vi "Generate Patch Seq Img Core.vi"(0 "tdms file ref":refnum<k34>, 1 "Channel to process":enum16{"Red", "Green"}(ring), 5 "All header parameters":T1={"Imaging Protocol"=enum."AOL Z-Stack", "Number of POI"=0, "Number of Miniscans"=0, "Number of Trials"=0, "Number of Cycles "=0, "# Averaged Frames"=0, "Laser power (%)"=0, "Pockels"=0.0, "Acquisition Length (sec)"=0.0, "Fill time (us)"=0.0, "POI Dwell time (us)"=0.0, "Miniscan Dwell time per pixel (us)"=0.0, "PMT 1"=0.0, "PMT 2"=0.0, "Back Apperture"=0.0, "Zoom"=0.0, "Frame Size"=200, "Center Frequency"=0.0, "Field of View"=0.0, "DwellTime (us)"=0.0, "Wavelength (nm)"=0.0, "AOL Z"=0.0, "AOL Mode"=enum."Raster", "GridXY"=0.0, "GridZ"=0.0, "TriggerDelay (sec)"=0.0, "Number of Pixels in Miniscan"=0, "Experiment folder path"=path "", "X centre"=0.0, "Y centre"=0.0, "Angle (degrees)"=0.0, "Plane Mode"=0, "Software version"=0.0, "Objective"="Olympus  20X", "MotorZ Calibration"=0, "Pockels Calibration"=0, "Threshold"=[], "Video length (sec)"=0.0, "Frame rate (fps)"=0, "Rectangle ROI length (pixels)"=0, "Rectangle ROI height (pixels)"=0} {"Pockels" format="%#.6g"; "Software version" format="%#.6g"; "Plane Mode" items=["XY Plane"]; "Angle (degrees)" format="%#.6g"; "Frame Size" items=["100X100"=100, "128X128"=128, "200X200"=200, "256X256"=256, "512X512"=512, "1024x1024"=1024, "2048x2048"=2048]; "Back Apperture" format="%#.6g"; "PMT 2" format="%#.6g"; "PMT 1" format="%#.6g"; "Miniscan Dwell time per pixel (us)" format="%#.6g"; "Zoom" format="%#.6g"; "POI Dwell time (us)" format="%#.6g"; "Acquisition Length (sec)" format="%#.6g"; "Fill time (us)" format="%#.6g"}, 7 "TDMS file path & name":path=path "C:/Users/Theo/Desktop/Datasets/140401_17_44_08-rig 3 debugging/Functional imaging TDMS data files/001.tdms", 9 "Patch Image Folder":path[](array[path]), 11 "error in (no error)":errorcluster, 13 "TIFF file handles":i32[](array[numeric]), 14 "Trial Number":i32) -> (4 "tdms file out":refnum<k34>, 15 "error out":errorcluster)   [LabVIEW 2013]
uses:
  User Interface/Visualisation/Functional Imaging Viewer/SubVIs/Experiment header interface/Typedefs/Header parameters cluster-ALL.ctl
  Typedefs/Imaging Protocols enum.ctl
  Typedefs/Frame Size.ctl
  Typedefs/AOL modes.ctl
  Typedefs/Plane Mode.ctl
  Typedefs/Objective selector control enum.ctl
  Typedefs/Channel Selector.ctl
  Globals/gl_funct TIFF export globals.vi
  <vilib>/vision/NI_Vision_Development_Module.lvlib
panel:
  out "Loop time (ms)":u32
  # "Re-entrant"
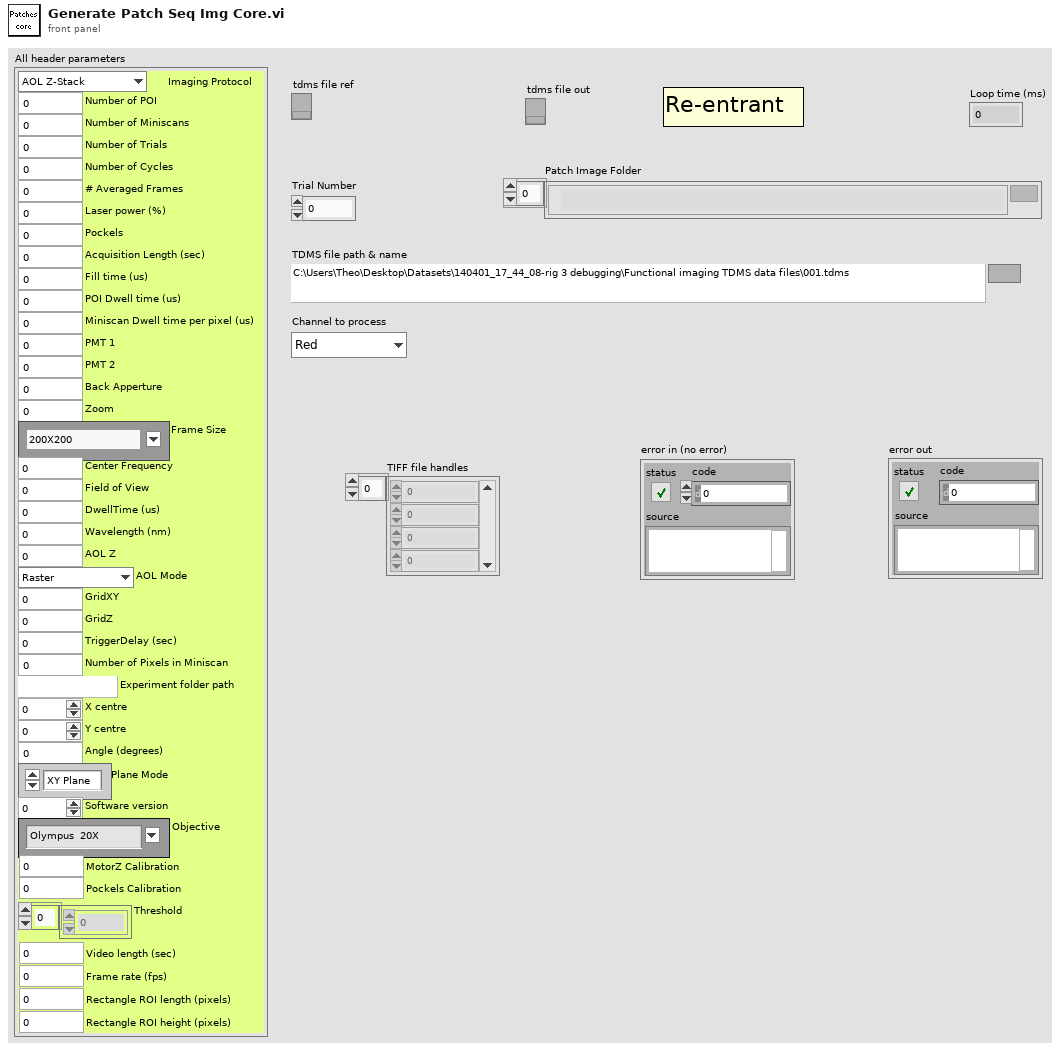
[diagram p1: front panel]
types:
  T1 = typedef "Header parameters cluster-ALL.ctl" = cluster{"Imaging Protocol":T2, "Number of POI":u16, "Number of Miniscans":u16, "Number of Trials":u16, "Number of Cycles ":u64, "# Averaged Frames":u16, "Laser power (%)":u8, "Pockels":dbl, "Acquisition Length (sec)":dbl, "Fill time (us)":dbl, "POI Dwell time (us)":dbl, "Miniscan Dwell time per pixel (us)":dbl, "PMT 1":dbl, "PMT 2":dbl, "Back Apperture":dbl, "Zoom":dbl, "Frame Size":T3, "Center Frequency":dbl, "Field of View":dbl, "DwellTime (us)":dbl, "Wavelength (nm)":dbl, "AOL Z":dbl, "AOL Mode":T4, "GridXY":dbl, "GridZ":dbl, "TriggerDelay (sec)":dbl, "Number of Pixels in Miniscan":u16, "Experiment folder path":path, "X centre":dbl, "Y centre":dbl, "Angle (degrees)":dbl, "Plane Mode":T5, "Software version":dbl, "Objective":T6, "MotorZ Calibration":u32, "Pockels Calibration":u32, "Threshold":u16[], "Video length (sec)":dbl, "Frame rate (fps)":u8, "Rectangle ROI length (pixels)":u16, "Rectangle ROI height (pixels)":u16}
  T2 = typedef "Imaging Protocols enum.ctl" = enum16{"AOL Z-Stack", "Motor Z Stack", "Functional Acquisition", "Single Plane Acquisition", "Volume Acquisition", "Live Imaging", "Live Plane Imaging", "Live Volume Imaging"}
  T3 = typedef "Frame Size.ctl" = u16
  T4 = typedef "AOL modes.ctl" = enum16{"Raster", "Structural", "Pointing", "Mini Scan", "Alignment"}
  T5 = typedef "Plane Mode.ctl" = u16
  T6 = typedef "Objective selector control enum.ctl" = string
  T7 = typedef "Funct TIFF exporter ctrl refs.ctl" = cluster{"This VI":refnum<vi>, "Current Experiment":refnum<vi>, "Imaging protocol":refnum<vi>, "Predominant ROI type":refnum<vi>, "Patches in Experiment":refnum<vi>, "Folder Path":refnum<vi>, "Export":refnum<vi>, "Trial number":refnum<vi>, "Output TIFF type":refnum<vi>}
  T8 = typedef "Exported TIFF type.ctl" = enum16{"One multi-page TIFF file for each rectangle", "Individual TIFF files"}
  T9 = typedef "Channel Selector.ctl" = enum16{"Red Channel", "Green Channel", "Blended"}
  T10 = cluster{"Number of cycles":i32, "number of planes":i32, "number of miniscans in a Plane":i32, "number of pixels in a miniscan":i32}
  T11 = typedef "Image Type" = u32
  T12 = typedef "IMAQ Image.ctl" = refnum<image>
  T13 = typedef "IMAQ AVI2 Refnum.ctl" = refnum<k20>
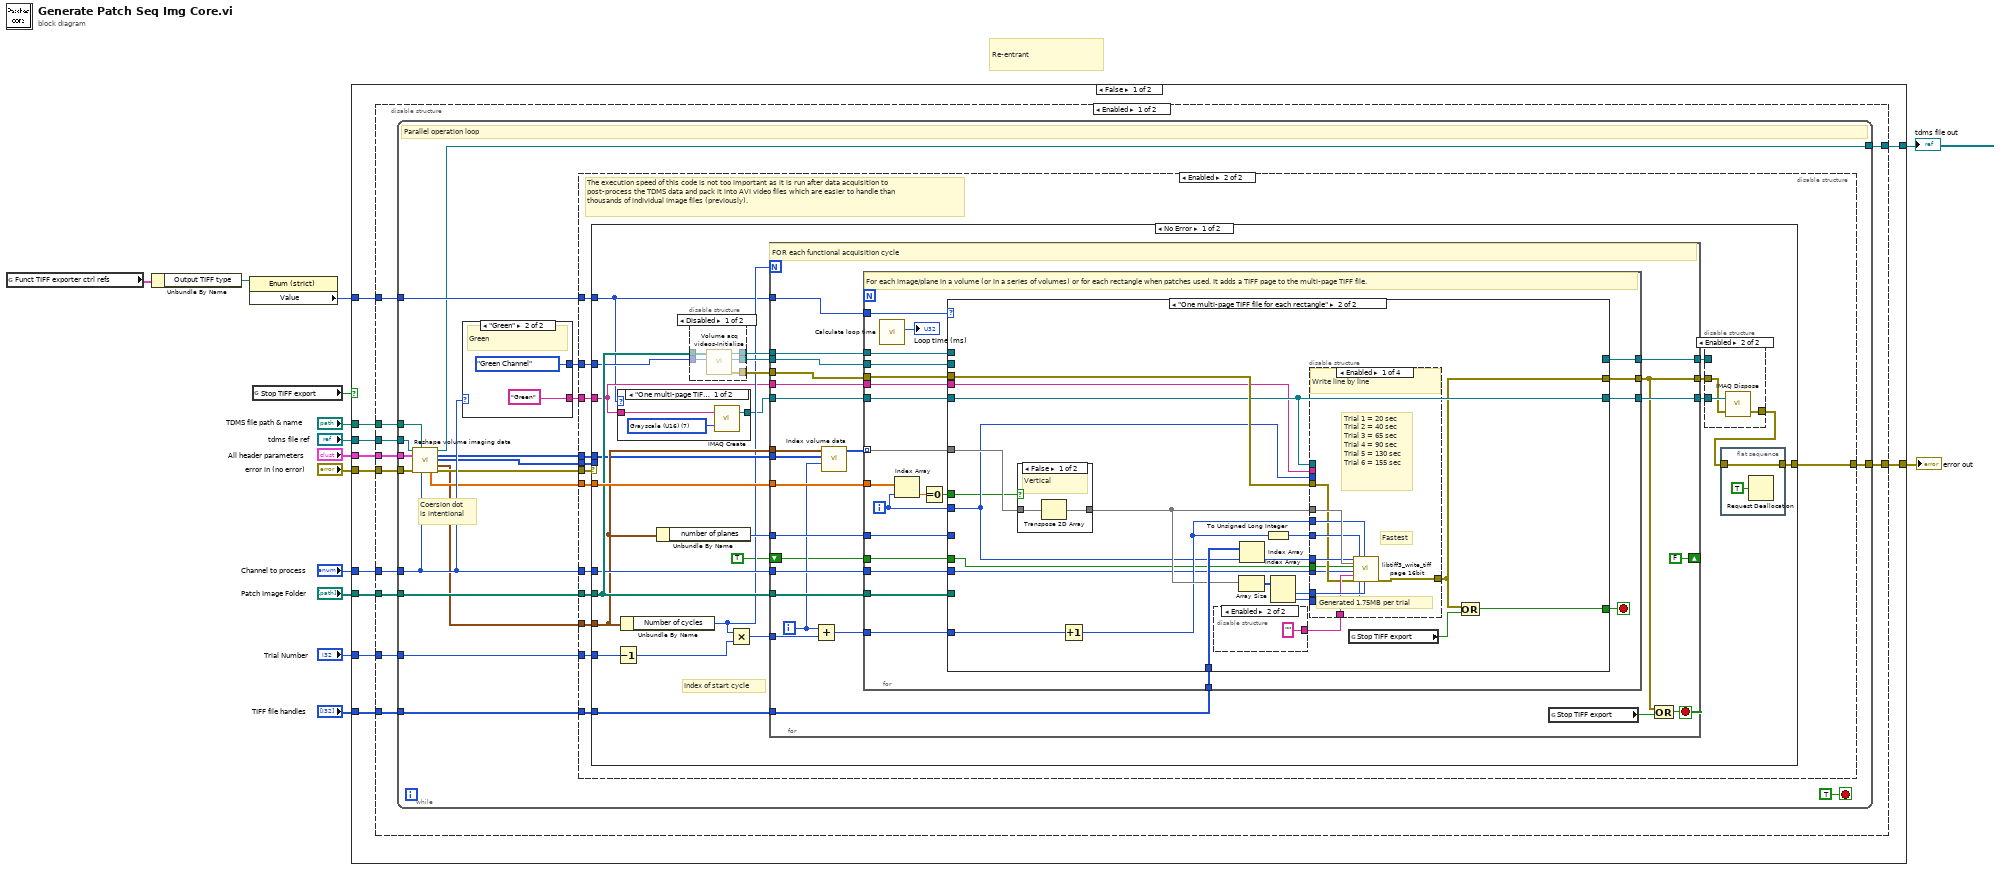
[diagram p0: block diagram]
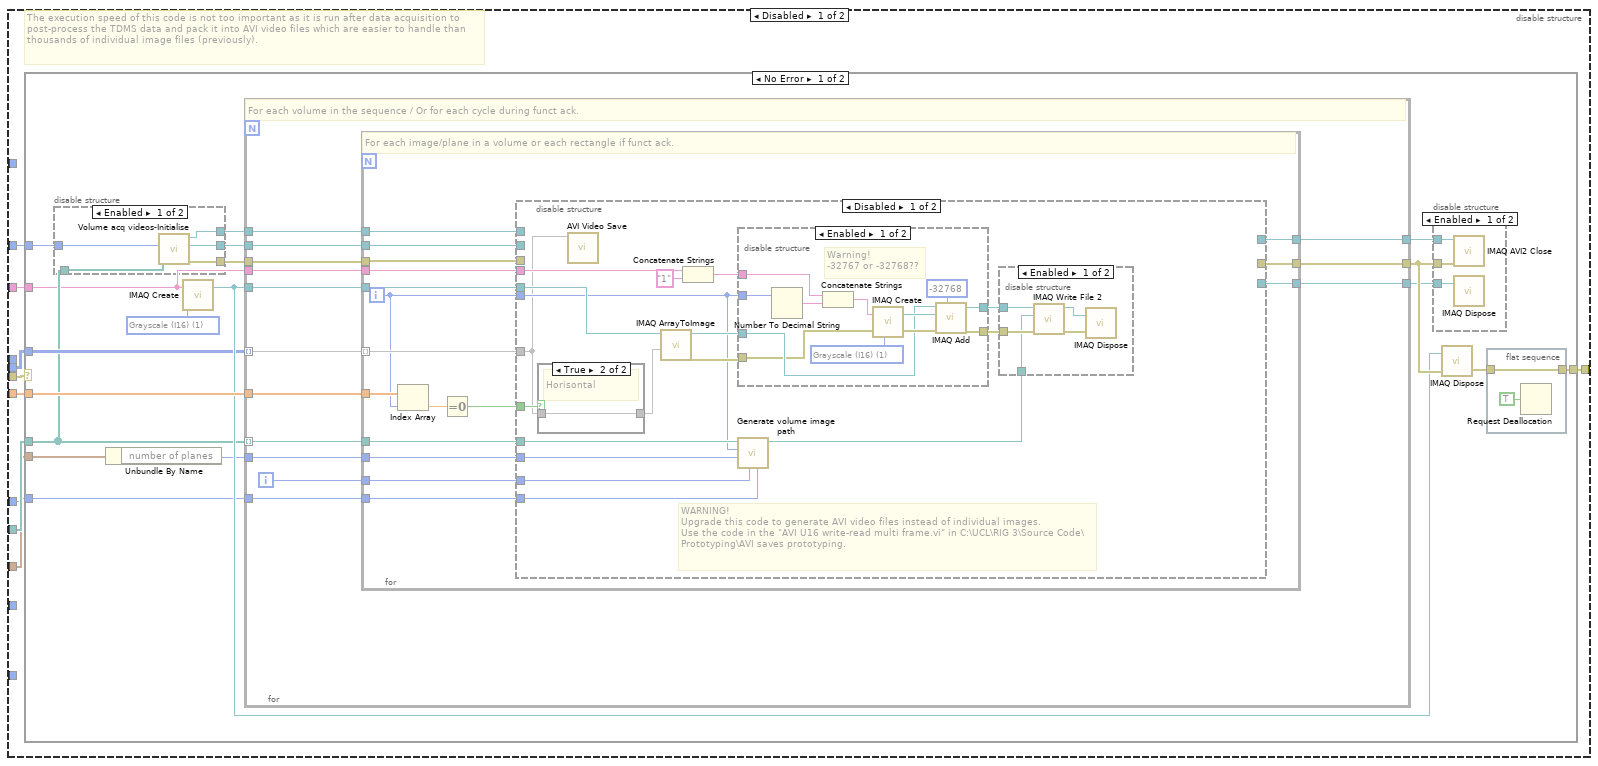
[diagram p2: hidden frame]
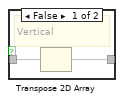
[diagram p5: hidden frame]
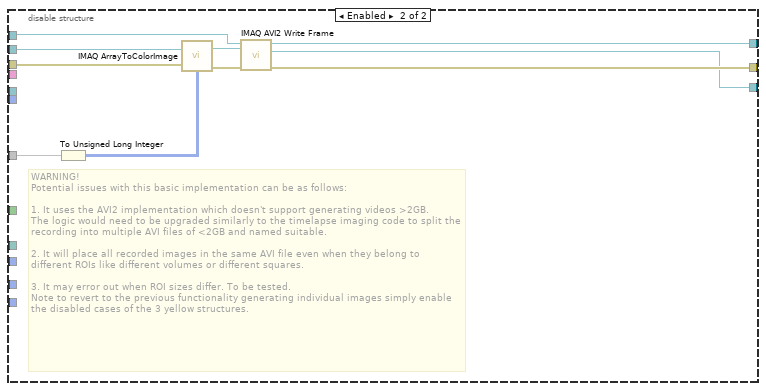
[diagram p8: hidden frame]
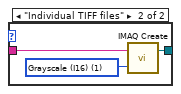
[diagram p10: hidden frame]
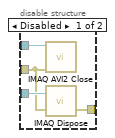
[diagram p12: hidden frame]
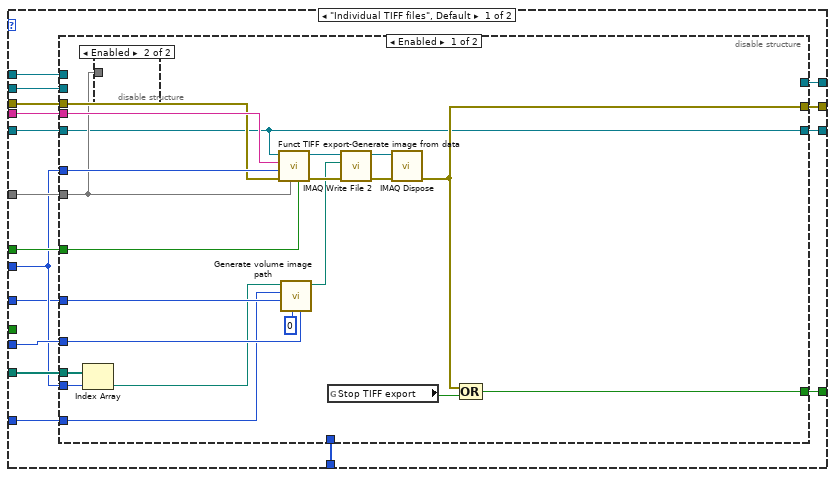
[diagram p13: hidden frame]
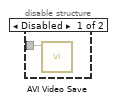
[diagram p14: hidden frame]
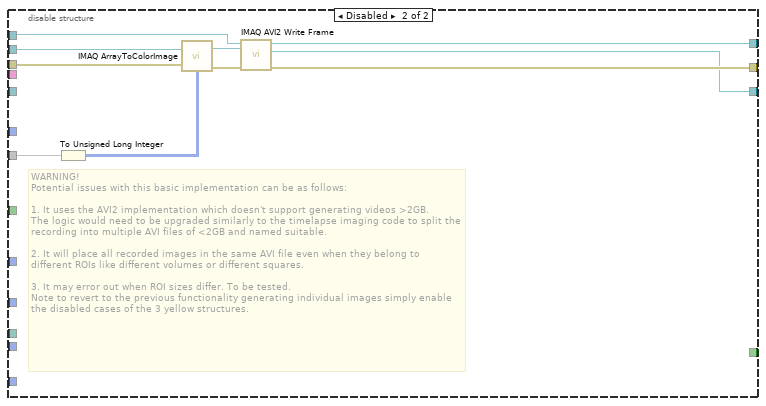
[diagram p15: hidden frame]
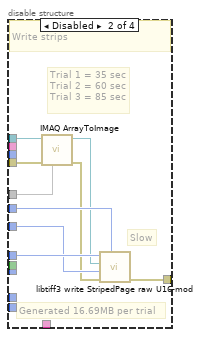
[diagram p16: hidden frame]
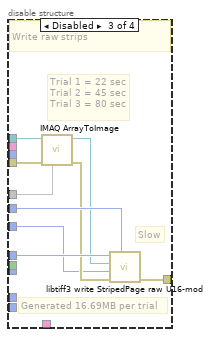
[diagram p17: hidden frame]
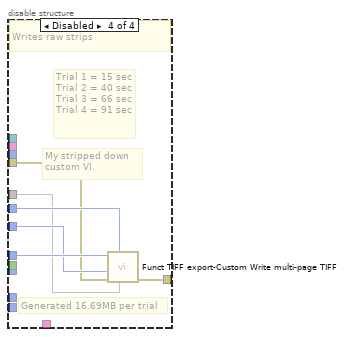
[diagram p18: hidden frame]
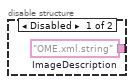
[diagram p19: hidden frame]
diagram:
  # "Re-entrant"
  n1 = global read "gl_funct TIFF export globals.vi" "Funct TIFF exporter ctrl refs"() -> (w6:T7)
  n2 = Unbundle By Name(w6) -> ("Output TIFF type"=w7:refnum<vi>)
  n3 = property on="Property Node" class="Enum (strict)"(reference=w7) -> ("Value"=w5:T8)  [unwired: 1 in, 2 out]
  n4 = global read "gl_funct TIFF export globals.vi" "Stop TIFF export"() -> (w10:bool)
  n5 = case shown="False" w10 {
    tunnel: [w25 w528] -> w14
    tunnel: "error in (no error)" -> [w24 w528]
    tunnel: "Channel to process" -> [w23 _]
    tunnel: "Patch Image Folder" -> [w22 _]
    tunnel: "Trial Number" -> [w21 _]
    tunnel: "TIFF file handles" -> [w20 _]
    tunnel: w5 -> [w19 _]
    tunnel: "tdms file ref" -> [w18 w527]
    tunnel: "All header parameters" -> [w17 _]
    tunnel: "TDMS file path & name" -> [w16 _]
    tunnel: [w15 w527] -> w1
    frame False {
      n6 = disable-structure shown="Enabled" {
        disable-tunnel: [w36 w399] -> w25
        disable-tunnel: w22 -> [w35 w398]
        disable-tunnel: w24 -> [w34 w397]
        disable-tunnel: w23 -> [w33 w396]
        disable-tunnel: w21 -> [w32 _]
        disable-tunnel: w20 -> [w31 _]
        disable-tunnel: w19 -> [w30 _]
        disable-tunnel: w18 -> [w29 w394]
        disable-tunnel: w17 -> [w28 w393]
        disable-tunnel: w16 -> [w27 w395]
        disable-tunnel: [w26 w392] -> w15
        frame Enabled {
          n7 = while {
            tunnel: [w55] -> w36
            tunnel: w35 -> [w54]
            tunnel: w34 -> [w53]
            tunnel: w33 -> [w52]
            tunnel: w32 -> [w51]
            tunnel: w31 -> [w50]
            tunnel: w30 -> [w49]
            tunnel: w29 -> [w38]
            tunnel: w28 -> [w41]
            tunnel: w27 -> [w40]
            tunnel: [w39] -> w26
            stop <- TRUE stop-if-true
            # "Coersion dot\nis intentional"
            # "Parallel operation loop"
            n8 = call "Reshape volume imaging data.vi"("tdms file ref"=w38, "TDMS file path & name"=w40, "All header parameters"=w41, "error in (no error)"=w53, "Channel to process"=w52) -> ("tdms file out"=w39:refnum<k34>, "Single channel data"=w43:u16[], "Channel 4D data"=w42:u16[][][][], "Volumetric parameters"=w44:T10, "Angles (deg)"=w45:dbl[], "error out"=w47:errorcluster)  [unwired: 5 in]
            n9 = case shown="\"Green\"" w52 {
              tunnel: ["Red" ("Image Name") "Green" ("Image Name")] -> w48
              tunnel: [Channel_Selector."Red Channel" ("Channel") Channel_Selector."Green Channel" ("Channel")] -> w46
              frame "Red", Default {
                # "Red"
              }
              frame "Green" {
                # "Green"
              }
            }
            n10 = disable-structure shown="Enabled" {
              disable-tunnel: [w64 w186] -> w55
              disable-tunnel: w54 -> [w63 w185]
              disable-tunnel: w48 -> [w62 w184]
              disable-tunnel: w42 -> [w61 w183]
              disable-tunnel: w47 -> [w60 w182]
              disable-tunnel: w46 -> [w59 w181]
              disable-tunnel: w45 -> [w58 w180]
              disable-tunnel: w52 -> [w57 w179]
              disable-tunnel: w44 -> [w56 w178]
              disable-tunnel: w43 -> [_ w177]
              disable-tunnel: w51 -> [_ w175]
              disable-tunnel: w50 -> [_ w176]
              disable-tunnel: w49 -> [_ w174]
              frame Disabled {
                # "The execution speed of this code is not too important as it is run after data acquisition to post-process the TDMS data and pack it into AVI video files which are easier to handle than thousands of individual image files (previously)."
                n11 = case shown="No Error" w60 {
                  selector: w60 -> [_ w173]
                  tunnel: [w68 w173] -> w64
                  tunnel: w58 -> [w82 _]
                  tunnel: w61 -> [w74 _]
                  tunnel: w56 -> [w65 _]
                  tunnel: w63 -> [w71 _]
                  tunnel: w62 -> [w70 _]
                  tunnel: w57 -> [w67 _]
                  tunnel: w59 -> [w66 _]
                  frame No Error {
                    w73 = T11 1 items=["Grayscale (U8)", "Grayscale (I16)", "Grayscale (SGL)", "Complex (CSG)", "RGB (U32)", "HSL (U32)", "RGB (U64)", "Grayscale (U16)"] ("Image Type")
                    n12 = disable-structure "Diagram Disable Structure" shown="Enabled" {
                      disable-tunnel: [w89 _] -> w75
                      disable-tunnel: [w88 _] -> w76
                      disable-tunnel: [w87 _] -> w77
                      disable-tunnel: w71 -> [w86 _]
                      disable-tunnel: w66 -> [w85 _]
                      frame Enabled {
                        n13 = call "Volume acq videos-Initialise.vi"("Channel"=w85, "created path"=w86) -> ("error out"=w89:errorcluster, "Temp Image"=w88:T12, "Refnum out"=w87:T13)  [unwired: 7 in]
                      }
                      frame Disabled {
                      }
                    }
                    n14 = Unbundle By Name(w65) -> ("number of planes"=w72:i32)
                    n15 = call "IMAQ Create"("Image Name"=w70, "Image Type"=w73) -> ("New Image"=w80:T12)  [unwired: 3 in, 1 out]
                    n16 = for {
                      tunnel: w74 -> [w106] mode=indexing
                      tunnel: w80 -> [w105]
                      tunnel: w71 -> [w104] mode=indexing
                      tunnel: w72 -> [w102]
                      tunnel: w76 -> [w101]
                      tunnel: w77 -> [w100]
                      tunnel: w75 -> [w99]
                      tunnel: [w98] -> w81
                      tunnel: [w97] -> w78
                      tunnel: [w96] -> w79
                      tunnel: w82 -> [w95]
                      tunnel: w70 -> [w94]
                      tunnel: w67 -> [w93]
                      i -> [w103]
                      # "For each volume in the sequence / Or for each cycle during funct ack."
                      n17 = for {
                        tunnel: w106 -> [w110] mode=indexing
                        tunnel: w105 -> [w123]
                        tunnel: w104 -> [w122]
                        tunnel: w103 -> [w121]
                        tunnel: w102 -> [w120]
                        tunnel: w101 -> [w118]
                        tunnel: w100 -> [w119]
                        tunnel: w99 -> [w117]
                        tunnel: [w116] -> w98
                        tunnel: [w115] -> w97
                        tunnel: [w114] -> w96
                        tunnel: w95 -> [w109]
                        tunnel: w94 -> [w112]
                        tunnel: w93 -> [w111]
                        i -> [w108]
                        # "For each image/plane in a volume or each rectangle if funct ack."
                        n18 = Index Array(array=w109, index=w108) -> (element=w107:dbl)
                        n19 = Equal To 0?(x=w107) -> (x = 0?=w113:bool)
                        n20 = disable-structure shown="Disabled" {
                          disable-tunnel: w123 -> [w140 _]
                          disable-tunnel: w122 -> [w135 _]
                          disable-tunnel: w121 -> [w133 _]
                          disable-tunnel: w120 -> [w132 _]
                          disable-tunnel: w108 -> [w131 _]
                          disable-tunnel: w119 -> [_ w169]
                          disable-tunnel: w118 -> [_ w168]
                          disable-tunnel: w117 -> [_ w167]
                          disable-tunnel: [_ w166] -> w116
                          disable-tunnel: [_ w165] -> w115
                          disable-tunnel: [_ w164] -> w114
                          disable-tunnel: w113 -> [w130 _]
                          disable-tunnel: w110 -> [w125 w163]
                          disable-tunnel: w112 -> [w128 _]
                          disable-tunnel: w111 -> [w124 _]
                          frame Disabled {
                            # "WARNING!\nUpgrade this code to generate AVI video files instead of individual images.\nUse the code in the \"AVI U16 write-read multi frame.vi\" in C:\\UCL\\RIG 3\\Source Code\\Prototyping\\AVI saves prototyping."
                            n21 = case shown="True" w130 {
                              tunnel: w125 -> [w142 w143]
                              tunnel: [w141 w143] -> w129
                              frame False {
                                # "Vertical"
                                n22 = Transpose 2D Array(2D array=w142) -> (transposed array=w141:u16[][])
                              }
                              frame True {
                                # "Horisontal"
                              }
                            }
                            n23 = call "AVI Video Save.vi"("Image Pixels"=w125) -> ()  [unwired: 9 in, 2 out]
                            n24 = call "IMAQ ArrayToImage"("Image Pixels (I16)"=w129, "Image"=w140) -> ("error out"=w136:errorcluster, "Image Out"=w139:T12)  [unwired: 8 in]
                            n25 = Concatenate Strings(w128, "1" ("string")) -> (w126:string)
                            n26 = call "Generate volume image path.vi"("Channel to process"=w124, "Volume index"=w133, "Number of planes"=w132, "Plane index (within its volume)"=w131, "Folder path"=w135) -> ("File path"=w134:path)  [unwired: 5 in, 1 out]
                            n27 = disable-structure shown="Enabled" {
                              disable-tunnel: w131 -> [w154 _]
                              disable-tunnel: w139 -> [w153 w162]
                              disable-tunnel: [w152 w162] -> w138
                              disable-tunnel: [w150 w161] -> w137
                              disable-tunnel: w136 -> [w151 w161]
                              disable-tunnel: w126 -> [w149 _]
                              frame Enabled {
                                w156 = T11 1 items=["Grayscale (U8)", "Grayscale (I16)", "Grayscale (SGL)", "Complex (CSG)", "RGB (U32)", "HSL (U32)", "RGB (U64)"] ("Image Type")
                                # "Warning!\n-32767 or -32768??"
                                n28 = Number To Decimal String(number=w154) -> (decimal integer string=w157:string)  [unwired: 1 in]
                                n29 = Concatenate Strings(w149, w157) -> (w158:string)
                                n30 = call "IMAQ Create"("Image Name"=w158, "Image Type"=w156, "error in (no error)"=w151) -> ("New Image"=w159:T12, "error out"=w160:errorcluster)  [unwired: 2 in]
                                n31 = call "IMAQ Add"("Image Src A"=w153, "Constant"=i16 -32768, "Image Dst"=w159, "error in (no error)"=w160) -> ("Image Dst Out"=w152:T12, "error out"=w150:errorcluster)  [unwired: 3 in]
                              }
                              frame Disabled {
                              }
                            }
                            n32 = disable-structure shown="Enabled" {
                              disable-tunnel: w138 -> [w146 _]
                              disable-tunnel: w137 -> [w145 _]
                              disable-tunnel: w134 -> [w144 _]
                              frame Enabled {
                                n33 = call-poly "IMAQ Write File 2"("error in (no error)"=w145, "File Path"=w144, "Image"=w146) -> ("error out"=w148:errorcluster, "Image Out (duplicate)"=w147:T12)  [unwired: 7 in]
                                n34 = call "IMAQ Dispose"("Image"=w147, "error in (no error)"=w148) -> ()  [unwired: 4 in, 1 out]
                              }
                              frame Disabled {
                              }
                            }
                          }
                          frame Enabled {
                            # "WARNING!\nPotential issues with this basic implementation can be as follows:\n\n1. It uses the AVI2 implementation which doesn't support generating videos >2GB. \nThe logic would need to be upgraded similarly to the timelapse imaging code to split the recording into multiple AVI files of <2GB and named suitable.\n\n2. It will place all recorded images in the same AVI file even when they belong to different ROIs like different volumes or different squares.\n\n3. It may error out when ROI sizes differ. To be tested.\nNote to revert to the previous functionality generating individual images simply enable the disabled cases of the 3 yellow structures."
                            n35 = To Unsigned Long Integer(number=w163) -> (unsigned 32bit integer=w171:u32[][])
                            n36 = call "IMAQ ArrayToColorImage"("Image Pixels (U32)"=w171, "Image"=w168, "error in (no error)"=w167) -> ("Image Out"=w172:T12, "error out"=w170:errorcluster)  [unwired: 1 in, 1 out]
                            n37 = call "IMAQ AVI2 Write Frame"("error in (no error)"=w170, "Image"=w172, "AVI Refnum"=w169) -> ("error out"=w166:errorcluster, "Image Out (duplicate)"=w164:T12, "AVI Refnum (duplicate)"=w165:T13)  [unwired: 6 in]
                          }
                        }
                      }
                    }
                    n38 = disable-structure "Diagram Disable Structure" shown="Enabled" {
                      disable-tunnel: w78 -> [w92 _]
                      disable-tunnel: w81 -> [w91 _]
                      disable-tunnel: w79 -> [w90 _]
                      frame Enabled {
                        n39 = call "IMAQ AVI2 Close"("error in (no error)"=w91, "AVI Refnum"=w92) -> ()  [unwired: 9 in, 1 out]
                        n40 = call "IMAQ Dispose"("Image"=w90) -> ()  [unwired: 5 in, 1 out]
                      }
                      frame Disabled {
                      }
                    }
                    n41 = call "IMAQ Dispose"("Image"=w80, "error in (no error)"=w81) -> ("error out"=w69:errorcluster)  [unwired: 4 in]
                    n42 = flat-sequence {
                      tunnel: w69 -> [w83]
                      tunnel: [w83] -> w68
                      frame #0 {
                        n43 = Request Deallocation(TRUE ("flag")) -> ()
                      }
                    }
                  }
                  frame Error {
                  }
                }
              }
              frame Enabled {
                # "The execution speed of this code is not too important as it is run after data acquisition to post-process the TDMS data and pack it into AVI video files which are easier to handle than thousands of individual image files (previously)."
                n44 = case shown="No Error" w182 {
                  selector: w182 -> [_ w387]
                  tunnel: [w202 w387] -> w186
                  tunnel: w180 -> [w210 _]
                  tunnel: w183 -> [_ _]
                  tunnel: w178 -> [w199 _]
                  tunnel: w185 -> [w203 _]
                  tunnel: w184 -> [w190 _]
                  tunnel: w179 -> [w201 _]
                  tunnel: w181 -> [w200 _]
                  tunnel: w177 -> [w198 _]
                  tunnel: w175 -> [w196 _]
                  tunnel: w176 -> [w195 _]
                  tunnel: w174 -> [w188 _]
                  frame No Error {
                    # "Index of start cycle"
                    n45 = Decrement(x=w196) -> (x-1=w194:i32)
                    n46 = case shown="\"One multi-page TIFF file for each rectangle\"" w188 {
                      tunnel: w190 -> [w212 w215]
                      tunnel: [w211 w214] -> w189
                      frame "One multi-page TIFF file for each rectangle" {
                        w213 = T11 7 items=["Grayscale (U8)", "Grayscale (I16)", "Grayscale (SGL)", "Complex (CSG)", "RGB (U32)", "HSL (U32)", "RGB (U64)", "Grayscale (U16)"] ("Image Type")
                        n47 = call "IMAQ Create"("Image Name"=w212, "Image Type"=w213) -> ("New Image"=w211:T12)  [unwired: 3 in, 1 out]
                      }
                      frame "Individual TIFF files" {
                        w216 = T11 1 items=["Grayscale (U8)", "Grayscale (I16)", "Grayscale (SGL)", "Complex (CSG)", "RGB (U32)", "HSL (U32)", "RGB (U64)", "Grayscale (U16)"] ("Image Type")
                        n48 = call "IMAQ Create"("Image Name"=w215, "Image Type"=w216) -> ("New Image"=w214:T12)  [unwired: 3 in, 1 out]
                      }
                    }
                    n49 = Unbundle By Name(w199) -> ("Number of cycles"=w191:i32)
                    n50 = Unbundle By Name(w199) -> ("number of planes"=w204:i32)
                    n51 = disable-structure shown="Disabled" {
                      disable-tunnel: [w221 _] -> w207
                      disable-tunnel: [w220 _] -> w206
                      disable-tunnel: [w219 _] -> w205
                      disable-tunnel: w203 -> [w218 _]
                      disable-tunnel: w200 -> [w217 _]
                      frame Disabled {
                        n52 = call "Volume acq videos-Initialise.vi"("Channel"=w217, "created path"=w218) -> ("error out"=w219:errorcluster, "Temp Image"=w220:T12, "Refnum out"=w221:T13)  [unwired: 7 in]
                      }
                      frame Enabled {
                      }
                    }
                    n53 = Multiply(x=w191, y=w194) -> (x*y=w197:i32)
                    n54 = for {
                      N: w191 -> [_]
                      tunnel: w189 -> [w254]
                      tunnel: w203 -> [w253]
                      tunnel: w204 -> [w252]
                      tunnel: w206 -> [w251]
                      tunnel: w207 -> [w250]
                      tunnel: w205 -> [w249]
                      tunnel: [w233] -> w193
                      tunnel: [w248] -> w208
                      tunnel: [w247] -> w209
                      tunnel: w210 -> [w246]
                      tunnel: w190 -> [w245]
                      tunnel: w201 -> [w244]
                      tunnel: w199 -> [w242]
                      tunnel: w198 -> [w241]
                      tunnel: w197 -> [w238]
                      tunnel: w195 -> [w237]
                      tunnel: w188 -> [w234]
                      shift-right: [FALSE] -> _
                      shift-left: TRUE -> [w232]
                      i -> [w239]
                      stop <- w236 stop-if-true
                      # "FOR each functional acquisition cycle"
                      n55 = Add(x=w239, y=w238) -> (x+y=w240:i32)
                      n56 = call "Index volume data.vi"("Cycle index"=w239, "Single trial data (single channel)"=w241, "Parameters Cluster"=w242) -> ("3D"=w243:u16[][][])  [unwired: 5 in, 3 out]
                      n57 = for {
                        tunnel: w243 -> [w256] mode=indexing
                        tunnel: w254 -> [w276]
                        tunnel: w253 -> [w275]
                        tunnel: w252 -> [w261]
                        tunnel: w251 -> [w273]
                        tunnel: w250 -> [w274]
                        tunnel: w249 -> [w272]
                        tunnel: [w271] -> w233
                        tunnel: [w270] -> w248
                        tunnel: [w269] -> w247
                        tunnel: w246 -> [w265]
                        tunnel: w245 -> [w267]
                        tunnel: w244 -> [w266]
                        tunnel: w240 -> [w263]
                        tunnel: w237 -> [w259]
                        tunnel: w234 -> [w258]
                        tunnel: w232 -> [w255]
                        i -> [w262]
                        stop <- w260 stop-if-true
                        # "For each image/plane in a volume (or in a series of volumes) or for each rectangle when patches used. It adds a TIFF page to the multi-page TIFF file."
                        n58 = call <userlib>:"Calculate loop time.vi"() -> ("Loop time (ms)"=→"Loop time (ms)":u32)  [unwired: 11 in]
                        n59 = Index Array(array=w265, index=w262) -> (element=w264:dbl)
                        n60 = Equal To 0?(x=w264) -> (x = 0?=w268:bool)
                        n61 = case shown="\"One multi-page TIFF file for each rectangle\"" w258 {
                          tunnel: w276 -> [w293 w332]
                          tunnel: w275 -> [w292 _]
                          tunnel: w274 -> [w291 _]
                          tunnel: w273 -> [w290 _]
                          tunnel: w272 -> [w289 w333]
                          tunnel: [w288 w328] -> w271
                          tunnel: [w287 _] -> w270
                          tunnel: [w286 w332] -> w269
                          tunnel: w268 -> [w285 w329]
                          tunnel: w267 -> [w284 w331]
                          tunnel: w266 -> [w283 w327]
                          tunnel: w256 -> [w282 w338]
                          tunnel: w263 -> [w281 w339]
                          tunnel: w262 -> [w280 w330]
                          tunnel: w261 -> [w279 _]
                          tunnel: [w278 w346] -> w260
                          tunnel: w259 -> [w277 w345]
                          tunnel: w255 -> [_ w326]
                          frame "Individual TIFF files", Default {
                            n62 = disable-structure shown="Enabled" {
                              disable-tunnel: w293 -> [w294 _]
                              disable-tunnel: w292 -> [w307 _]
                              disable-tunnel: w279 -> [w312 _]
                              disable-tunnel: w280 -> [w311 _]
                              disable-tunnel: w291 -> [_ w322]
                              disable-tunnel: w290 -> [_ w321]
                              disable-tunnel: w289 -> [w297 w320]
                              disable-tunnel: [w303 w319] -> w288
                              disable-tunnel: [_ w318] -> w287
                              disable-tunnel: [w294 w317] -> w286
                              disable-tunnel: w285 -> [w296 _]
                              disable-tunnel: w282 -> [w295 w316]
                              disable-tunnel: w284 -> [w310 _]
                              disable-tunnel: w283 -> [w309 _]
                              disable-tunnel: w280 -> [w302 _]
                              disable-tunnel: w281 -> [w306 _]
                              disable-tunnel: [w304 _] -> w278
                              disable-tunnel: w277 -> [_ _]
                              frame Enabled {
                                n63 = Index Array(array=w307, index=w302) -> (element=w308:path)
                                n64 = disable-structure shown="Enabled" {
                                disable-tunnel: w295 -> [w315 _]
                                frame Disabled {
                                n65 = call "AVI Video Save.vi"("Image Pixels"=w315) -> ()  [unwired: 9 in, 2 out]
                                }
                                frame Enabled {
                                }
                                }
                                n66 = call "Funct TIFF export-Generate image from data.vi"("Horisontal (T)"=w296, "3D"=w295, "error in (no error)"=w297, "Rectangle index"=w311, "Image Name"=w310, "Refnum in"=w294) -> ("error out"=w313:errorcluster, "Refnum out"=w314:T12)  [unwired: 4 in]
                                n67 = call "Generate volume image path.vi"("Channel to process"=w309, "Volume index"=0, "Number of planes"=w312, "Plane index (within its volume)"=w306, "Folder path"=w308) -> ("File path"=w299:path)  [unwired: 5 in, 1 out]
                                n68 = global read "gl_funct TIFF export globals.vi" "Stop TIFF export"() -> (w305:bool)
                                n69 = call-poly "IMAQ Write File 2"("error in (no error)"=w313, "File Path"=w299, "Image"=w314) -> ("error out"=w301:errorcluster, "Image Out (duplicate)"=w300:T12)  [unwired: 7 in]
                                n70 = call "IMAQ Dispose"("Image"=w300, "error in (no error)"=w301) -> ("error out"=w303:errorcluster)  [unwired: 4 in]
                                n71 = Compound Arithmetic op=OR(w303, w305) -> (w304:bool)
                              }
                              frame Disabled {
                                # "WARNING!\nPotential issues with this basic implementation can be as follows:\n\n1. It uses the AVI2 implementation which doesn't support generating videos >2GB. \nThe logic would need to be upgraded similarly to the timelapse imaging code to split the recording into multiple AVI files of <2GB and named suitable.\n\n2. It will place all recorded images in the same AVI file even when they belong to different ROIs like different volumes or different squares.\n\n3. It may error out when ROI sizes differ. To be tested.\nNote to revert to the previous functionality generating individual images simply enable the disabled cases of the 3 yellow structures."
                                n72 = To Unsigned Long Integer(number=w316) -> (unsigned 32bit integer=w324:u32[][])
                                n73 = call "IMAQ ArrayToColorImage"("Image Pixels (U32)"=w324, "Image"=w321, "error in (no error)"=w320) -> ("Image Out"=w325:T12, "error out"=w323:errorcluster)  [unwired: 1 in, 1 out]
                                n74 = call "IMAQ AVI2 Write Frame"("error in (no error)"=w323, "Image"=w325, "AVI Refnum"=w322) -> ("error out"=w319:errorcluster, "Image Out (duplicate)"=w317:T12, "AVI Refnum (duplicate)"=w318:T13)  [unwired: 6 in]
                              }
                            }
                          }
                          frame "One multi-page TIFF file for each rectangle" {
                            n75 = case shown="False" w329 {
                              tunnel: w338 -> [w385 w386]
                              tunnel: [w384 w386] -> w344
                              frame False {
                                # "Vertical"
                                n76 = Transpose 2D Array(2D array=w385) -> (transposed array=w384:u16[][])
                              }
                              frame True {
                                # "Horisontal"
                              }
                            }
                            n77 = Increment(x=w339) -> (x+1=w336:i32)
                            n78 = disable-structure shown="Enabled" {
                              disable-tunnel: [w382 "" ("ImageDescription")] -> w340
                              frame Disabled {
                                w382 = "OME.xml.string"  # ImageDescription
                              }
                              frame Enabled {
                              }
                            }
                            n79 = Array Size(array=w344) -> (size(s)=w343:i32[])
                            n80 = Index Array(array=w345, index=w330) -> (element=w337:i32)
                            n81 = To Unsigned Long Integer(number=w336) -> (unsigned 32bit integer=w335:u32)
                            n82 = Index Array(array=w343) -> (element #1=w342:i32, element #2=w341:i32)  [unwired: 2 in]
                            n83 = disable-structure shown="Enabled" {
                              disable-tunnel: [w357 w359 w370 w378] -> w328
                              disable-tunnel: w344 -> [w356 w360 w373 w377]
                              disable-tunnel: w342 -> [w355 _ _ _]
                              disable-tunnel: w341 -> [w354 _ _ _]
                              disable-tunnel: w340 -> [w353 _ _ _]
                              disable-tunnel: w337 -> [w352 w365 w371 w380]
                              disable-tunnel: w336 -> [w351 w366 w372 w381]
                              disable-tunnel: w335 -> [w350 w364 w367 w379]
                              disable-tunnel: w333 -> [w349 w361 w374 w376]
                              disable-tunnel: w332 -> [_ w363 w375 _]
                              disable-tunnel: w331 -> [_ _ _ _]
                              disable-tunnel: w330 -> [_ _ _ _]
                              disable-tunnel: w327 -> [w348 _ _ _]
                              disable-tunnel: w326 -> [w347 _ _ _]
                              frame Enabled {
                                # "Trial 1 = 20 sec\nTrial 2 = 40 sec\nTrial 3 = 65 sec\nTrial 4 = 90 sec\nTrial 5 = 130 sec\nTrial 6 = 155 sec"
                                # "Fastest"
                                # "Generated 1.75MB per trial"
                                # "Write line by line"
                                n84 = call "libtiff3_write_tiff page 16bit.vi"("Handle"=w352, "Image Pixels (U16)"=w356, "Reset"=w347, "Channel to process"=w348, "ImageDescription"=w353, "error in (no error)"=w349, "page"=w350, "x.pixels"=w354, "totalpages"=w351, "y.pixels"=w355) -> ("error out"=w357:errorcluster)  [unwired: 8 in, 1 out]
                              }
                              frame Disabled {
                                # "Trial 1 = 35 sec\nTrial 2 = 60 sec\nTrial 3 = 85 sec"
                                # "Slow"
                                # "Generated 16.69MB per trial"
                                # "Write strips"
                                n85 = call "IMAQ ArrayToImage"("Image Pixels (U16)"=w360, "error in (no error)"=w361, "Image"=w363) -> ("error out"=w362:errorcluster, "Image Out"=w358:T12)  [unwired: 7 in]
                                n86 = call "libtiff3 write StripedPage raw U16-mod.vi"("totalpages"=w366, "error in (no error)"=w362, "page"=w364, "Image"=w358, "Handle"=w365) -> ("error out"=w359:errorcluster)  [unwired: 5 in, 1 out]
                              }
                              frame Disabled {
                                # "Slow"
                                # "Trial 1 = 22 sec\nTrial 2 = 45 sec\nTrial 3 = 80 sec"
                                # "Generated 16.69MB per trial"
                                # "Write raw strips"
                                n87 = call "IMAQ ArrayToImage"("Image Pixels (U16)"=w373, "error in (no error)"=w374, "Image"=w375) -> ("error out"=w369:errorcluster, "Image Out"=w368:T12)  [unwired: 7 in]
                                n88 = call "libtiff3 write StripedPage raw U16-mod.vi"("totalpages"=w372, "error in (no error)"=w369, "page"=w367, "Image"=w368, "Handle"=w371) -> ("error out"=w370:errorcluster)  [unwired: 5 in, 1 out]
                              }
                              frame Disabled {
                                # "My stripped down\ncustom VI."
                                # "Trial 1 = 15 sec\nTrial 2 = 40 sec\nTrial 3 = 66 sec\nTrial 4 = 91 sec"
                                # "Generated 16.69MB per trial"
                                # "Writes raw strips"
                                n89 = call "Funct TIFF export-Custom Write multi-page TIFF.vi"("Image Pixels (U16)"=w377, "totalpages"=w381, "error in (no error)"=w376, "page"=w379, "Handle"=w380) -> ("error out"=w378:errorcluster)  [unwired: 5 in, 1 out]
                              }
                            }
                            n90 = global read "gl_funct TIFF export globals.vi" "Stop TIFF export"() -> (w334:bool)
                            n91 = Compound Arithmetic op=OR(w328, w334) -> (w346:bool)
                          }
                        }
                      }
                      n92 = global read "gl_funct TIFF export globals.vi" "Stop TIFF export"() -> (w235:bool)
                      n93 = Compound Arithmetic op=OR(w233, w235) -> (w236:bool)
                    }
                    n94 = disable-structure "Diagram Disable Structure" shown="Enabled" {
                      disable-tunnel: w208 -> [w227 _]
                      disable-tunnel: w193 -> [w224 w229]
                      disable-tunnel: w209 -> [w226 w230]
                      disable-tunnel: [w225 w228] -> w192
                      frame Disabled {
                        n95 = call "IMAQ AVI2 Close"("error in (no error)"=w224, "AVI Refnum"=w227) -> ()  [unwired: 9 in, 1 out]
                        n96 = call "IMAQ Dispose"("Image"=w226, "error in (no error)"=w224) -> ("error out"=w225:errorcluster)  [unwired: 4 in]
                      }
                      frame Enabled {
                        n97 = call "IMAQ Dispose"("Image"=w230, "error in (no error)"=w229) -> ("error out"=w228:errorcluster)  [unwired: 4 in]
                      }
                    }
                    n98 = flat-sequence {
                      tunnel: w192 -> [w222]
                      tunnel: [w222] -> w202
                      frame #0 {
                        n99 = Request Deallocation(TRUE ("flag")) -> ()
                      }
                    }
                  }
                  frame Error {
                  }
                }
              }
            }
          }
        }
        frame Disabled {
          # "The While Loop causes all instances of this VI to execute in parallel. (While loop is REDUNDANT)"
          n100 = while {
            tunnel: [w413] -> w399
            tunnel: w398 -> [w412]
            tunnel: w395 -> [w402]
            tunnel: w397 -> [w409]
            tunnel: w393 -> [w406]
            tunnel: w396 -> [w403]
            tunnel: w394 -> [w401]
            tunnel: [w400] -> w392
            stop <- TRUE stop-if-true
            # "The execution speed of this code is not too important as it is run after data acquisition to post-process the TDMS data and pack it into AVI video files which are easier to handle than thousands of individual image files (previously)."
            n101 = call "Reshape volume imaging data.vi"("tdms file ref"=w401, "TDMS file path & name"=w402, "All header parameters"=w406, "error in (no error)"=w409, "Channel to process"=w403) -> ("tdms file out"=w400:refnum<k34>, "Volumetric parameters"=w404:T10, "Angles (deg)"=w405:dbl[], "error out"=w410:errorcluster)  [unwired: 5 in, 2 out]
            n102 = case shown="\"Green\"" w403 {
              tunnel: ["Red" ("Image Name") "Green" ("Image Name")] -> w411
              tunnel: [Channel_Selector."Red Channel" ("Channel") Channel_Selector."Green Channel" ("Channel")] -> w408
              frame "Red", Default {
                # "Red"
              }
              frame "Green" {
                # "Green"
              }
            }
            n103 = case shown="No Error" w410 {
              selector: w410 -> [_ w526]
              tunnel: [w420 w526] -> w413
              tunnel: w405 -> [w435 _]
              tunnel: w400 -> [w427 _]
              tunnel: w404 -> [w424 _]
              tunnel: w412 -> [w423 _]
              tunnel: w411 -> [w422 _]
              tunnel: w403 -> [w419 _]
              tunnel: w408 -> [w418 _]
              frame No Error {
                w426 = T11 1 items=["Grayscale (U8)", "Grayscale (I16)", "Grayscale (SGL)", "Complex (CSG)", "RGB (U32)", "HSL (U32)", "RGB (U64)", "Grayscale (U16)"] ("Image Type")
                n104 = disable-structure "Diagram Disable Structure" shown="Enabled" {
                  disable-tunnel: [w442 _] -> w428
                  disable-tunnel: [w441 _] -> w429
                  disable-tunnel: [w440 _] -> w430
                  disable-tunnel: w423 -> [w439 _]
                  disable-tunnel: w418 -> [w438 _]
                  frame Enabled {
                    n105 = call "Volume acq videos-Initialise.vi"("Channel"=w438, "created path"=w439) -> ("error out"=w442:errorcluster, "Temp Image"=w441:T12, "Refnum out"=w440:T13)  [unwired: 7 in]
                  }
                  frame Disabled {
                  }
                }
                n106 = Unbundle By Name(w424) -> ("number of planes"=w425:i32)
                n107 = call "IMAQ Create"("Image Name"=w422, "Image Type"=w426) -> ("New Image"=w433:T12)  [unwired: 3 in, 1 out]
                n108 = for {
                  tunnel: w427 -> [w459]
                  tunnel: w433 -> [w458]
                  tunnel: w423 -> [w457] mode=indexing
                  tunnel: w425 -> [w455]
                  tunnel: w429 -> [w454]
                  tunnel: w430 -> [w453]
                  tunnel: w428 -> [w452]
                  tunnel: [w451] -> w434
                  tunnel: [w450] -> w431
                  tunnel: [w449] -> w432
                  tunnel: w435 -> [w448]
                  tunnel: w422 -> [w447]
                  tunnel: w419 -> [w446]
                  i -> [w456]
                  # "For each volume in the sequence / Or for each cycle during funct ack."
                  n109 = for {
                    tunnel: w459 -> [w463]
                    tunnel: w458 -> [w476]
                    tunnel: w457 -> [w475]
                    tunnel: w456 -> [w474]
                    tunnel: w455 -> [w473]
                    tunnel: w454 -> [w471]
                    tunnel: w453 -> [w472]
                    tunnel: w452 -> [w470]
                    tunnel: [w469] -> w451
                    tunnel: [w468] -> w450
                    tunnel: [w467] -> w449
                    tunnel: w448 -> [w462]
                    tunnel: w447 -> [w465]
                    tunnel: w446 -> [w464]
                    i -> [w461]
                    # "For each image/plane in a volume or each rectangle if funct ack."
                    n110 = Index Array(array=w462, index=w461) -> (element=w460:dbl)
                    n111 = Equal To 0?(x=w460) -> (x = 0?=w466:bool)
                    n112 = disable-structure shown="Disabled" {
                      disable-tunnel: w476 -> [w493 _]
                      disable-tunnel: w475 -> [w488 _]
                      disable-tunnel: w474 -> [w486 _]
                      disable-tunnel: w473 -> [w485 _]
                      disable-tunnel: w461 -> [w484 _]
                      disable-tunnel: w472 -> [_ w522]
                      disable-tunnel: w471 -> [_ w521]
                      disable-tunnel: w470 -> [_ w520]
                      disable-tunnel: [_ w519] -> w469
                      disable-tunnel: [_ w518] -> w468
                      disable-tunnel: [_ w517] -> w467
                      disable-tunnel: w466 -> [w483 _]
                      disable-tunnel: w463 -> [w478 w516]
                      disable-tunnel: w465 -> [w481 _]
                      disable-tunnel: w464 -> [w477 _]
                      frame Disabled {
                        # "WARNING!\nUpgrade this code to generate AVI video files instead of individual images.\nUse the code in the \"AVI U16 write-read multi frame.vi\" in C:\\UCL\\RIG 3\\Source Code\\Prototyping\\AVI saves prototyping."
                        n113 = case shown="True" w483 {
                          tunnel: w478 -> [w495 w496]
                          tunnel: [w494 w496] -> w482
                          frame False {
                            # "Vertical"
                            n114 = Transpose 2D Array(2D array=w495) -> (transposed array=w494:refnum<k34>[][])
                          }
                          frame True {
                            # "Horisontal"
                          }
                        }
                        n115 = call "AVI Video Save.vi"("Image Pixels"=w478) -> ()  [unwired: 9 in, 2 out]
                        n116 = call "IMAQ ArrayToImage"("Image Pixels (I16)"=w482, "Image"=w493) -> ("error out"=w489:errorcluster, "Image Out"=w492:T12)  [unwired: 8 in]
                        n117 = Concatenate Strings(w481, "1" ("string")) -> (w479:string)
                        n118 = call "Generate volume image path.vi"("Channel to process"=w477, "Volume index"=w486, "Number of planes"=w485, "Plane index (within its volume)"=w484, "Folder path"=w488) -> ("File path"=w487:path)  [unwired: 5 in, 1 out]
                        n119 = disable-structure shown="Enabled" {
                          disable-tunnel: w484 -> [w507 _]
                          disable-tunnel: w492 -> [w506 w515]
                          disable-tunnel: [w505 w515] -> w491
                          disable-tunnel: [w503 w514] -> w490
                          disable-tunnel: w489 -> [w504 w514]
                          disable-tunnel: w479 -> [w502 _]
                          frame Enabled {
                            w509 = T11 1 items=["Grayscale (U8)", "Grayscale (I16)", "Grayscale (SGL)", "Complex (CSG)", "RGB (U32)", "HSL (U32)", "RGB (U64)"] ("Image Type")
                            # "Warning!\n-32767 or -32768??"
                            n120 = Number To Decimal String(number=w507) -> (decimal integer string=w510:string)  [unwired: 1 in]
                            n121 = Concatenate Strings(w502, w510) -> (w511:string)
                            n122 = call "IMAQ Create"("Image Name"=w511, "Image Type"=w509, "error in (no error)"=w504) -> ("New Image"=w512:T12, "error out"=w513:errorcluster)  [unwired: 2 in]
                            n123 = call "IMAQ Add"("Image Src A"=w506, "Constant"=i16 -32768, "Image Dst"=w512, "error in (no error)"=w513) -> ("Image Dst Out"=w505:T12, "error out"=w503:errorcluster)  [unwired: 3 in]
                          }
                          frame Disabled {
                          }
                        }
                        n124 = disable-structure shown="Enabled" {
                          disable-tunnel: w491 -> [w499 _]
                          disable-tunnel: w490 -> [w498 _]
                          disable-tunnel: w487 -> [w497 _]
                          frame Enabled {
                            n125 = call-poly "IMAQ Write File 2"("error in (no error)"=w498, "File Path"=w497, "Image"=w499) -> ("error out"=w501:errorcluster, "Image Out (duplicate)"=w500:T12)  [unwired: 7 in]
                            n126 = call "IMAQ Dispose"("Image"=w500, "error in (no error)"=w501) -> ()  [unwired: 4 in, 1 out]
                          }
                          frame Disabled {
                          }
                        }
                      }
                      frame Enabled {
                        # "WARNING!\nPotential issues with this basic implementation can be as follows:\n\n1. It uses the AVI2 implementation which doesn't support generating videos >2GB. \nThe logic would need to be upgraded similarly to the timelapse imaging code to split the recording into multiple AVI files of <2GB and named suitable.\n\n2. It will place all recorded images in the same AVI file even when they belong to different ROIs like different volumes or different squares.\n\n3. It may error out when ROI sizes differ. To be tested.\nNote to revert to the previous functionality generating individual images simply enable the disabled cases of the 3 yellow structures."
                        n127 = To Unsigned Long Integer(number=w516) -> (unsigned 32bit integer=w524:u32)
                        n128 = call "IMAQ ArrayToColorImage"("Image Pixels (U32)"=w524, "Image"=w521, "error in (no error)"=w520) -> ("Image Out"=w525:T12, "error out"=w523:errorcluster)  [unwired: 1 in, 1 out]
                        n129 = call "IMAQ AVI2 Write Frame"("error in (no error)"=w523, "Image"=w525, "AVI Refnum"=w522) -> ("error out"=w519:errorcluster, "Image Out (duplicate)"=w517:T12, "AVI Refnum (duplicate)"=w518:T13)  [unwired: 6 in]
                      }
                    }
                  }
                }
                n130 = disable-structure "Diagram Disable Structure" shown="Enabled" {
                  disable-tunnel: w431 -> [w445 _]
                  disable-tunnel: w434 -> [w444 _]
                  disable-tunnel: w432 -> [w443 _]
                  frame Enabled {
                    n131 = call "IMAQ AVI2 Close"("error in (no error)"=w444, "AVI Refnum"=w445) -> ()  [unwired: 9 in, 1 out]
                    n132 = call "IMAQ Dispose"("Image"=w443) -> ()  [unwired: 5 in, 1 out]
                  }
                  frame Disabled {
                  }
                }
                n133 = call "IMAQ Dispose"("Image"=w433, "error in (no error)"=w434) -> ("error out"=w421:errorcluster)  [unwired: 4 in]
                n134 = flat-sequence {
                  tunnel: w421 -> [w436]
                  tunnel: [w436] -> w420
                  frame #0 {
                    n135 = Request Deallocation(TRUE ("flag")) -> ()
                  }
                }
              }
              frame Error {
              }
            }
          }
        }
      }
    }
    frame True {
    }
  }
  "error out" <- w14
  "tdms file out" <- w1
